vi "SetFilePath.vi"(8 "error in (no error)":errorcluster, 10 "FilePath":path, 11 "DocumentClass in":refnum<class "Document.lvclass">) -> (0 "error out":errorcluster, 3 "DocumentClass out":refnum<class "Document.lvclass">)   [LabVIEW 2021, in "ProligentXMLGenerator.lvlib" / "Document.lvclass"]
doc: "The FileName is used to identify the type of document and should contain an extension so that the appropriate application is launched when the user requests to view the document content.\n\nLimited to 255 characters."
uses:
  Document.lvclass
  Document.lvclass/Document.ctl
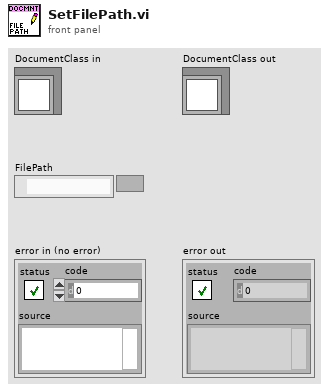
[diagram p1: front panel]
types:
  T1 = typedef "ProligentXMLGenerator.lvlib/Document.lvclass/Data.ctl" = cluster{"Name":string, "CustomData":refnum<class "CustomData.lvclass">, "Identifier":refnum<class "Guid.lvclass">, "NameType":refnum<class "NonEmptyString_255.lvclass">, "FileName":refnum<class "NonEmptyString_255.lvclass">, "Description":refnum<class "NonNullableString_600.lvclass">, "FilePath":path, "DestinationFolder":path}
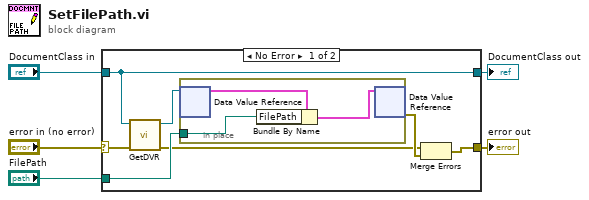
[diagram p0: block diagram]
diagram:
  n1 = case shown="No Error" "error in (no error)" {
    selector: "error in (no error)" -> [w10 w16]
    tunnel: "DocumentClass in" -> [w7 w17]
    tunnel: [w9 w16] -> w2
    tunnel: "FilePath" -> [w8 _]
    tunnel: [w7 w17] -> w4
    frame No Error {
      n2 = call "GetDVR.vi"("error in"=w10, "Document in"=w7) -> ("error out"=w6:errorcluster, "DVRReference"=w11:refnum<data-value>)  [unwired: 8 in]
      n3 = in-place "In Place Element Structure" {
        in-place-border: w8 -> [w13]
        n4 = in-place-dvr #1(w11) -> (w15:T1)  [unwired: 1 out]
        n5 = Bundle By Name(cluster=w15, "FilePath"=w13) -> (w14:T1)
        n6 = in-place-dvr #1(w14) -> (w12:errorcluster)  [unwired: 1 out]
      }
      n7 = Merge Errors(w6, w12) -> (w9:errorcluster)
    }
    frame Error {
    }
  }
  "error out" <- w2
  "DocumentClass out" <- w4
